vi "test.add.data.to.buffer.vi"() -> (3 "All Passed":bool=TRUE)   [LabVIEW 2020]
uses:
  data.ctl
  buffer.test.case.ctl
panel:
  in  "Test Case #12 - Buffer has 16 elements, Data has 3 elements":T1={"data.valid"=TRUE, "data"={"enabled"=[TRUE, TRUE, TRUE, FALSE, FALSE, FALSE, FALSE, FALSE], "byte"=[1, 2, 3, 4, 5, 6, 7, 0]}, "buffer"=[1234605616436508552, 48057234611961600, 0, 0, 0, 0, 0, 0, 0], "buffer.length"=16, "exp.buffer.value.1"=72623842526232576, "index 1"=2, "exp.buffer.value.2"=0, "index 2"=3, "exp.buffer.length"=19} {"exp.buffer.value.2" format="%.0x"; "index 1" format="%.0x"; "exp.buffer.value.1" format="%.0x"; "buffer" format="%.0x"; "data"."byte" format="%.0x"}
  out "Passed 12":bool=TRUE
  in  "Test Case #11 - Buffer has 16 elements, Data has 8 elements":T1={"data.valid"=TRUE, "data"={"enabled"=[TRUE, TRUE, TRUE, TRUE, TRUE, TRUE, TRUE, TRUE], "byte"=[1, 2, 3, 4, 5, 6, 7, 8]}, "buffer"=[1234605616436508552, 48057234611961600, 0, 0, 0, 0, 0, 0, 0], "buffer.length"=16, "exp.buffer.value.1"=72623859790382856, "index 1"=2, "exp.buffer.value.2"=0, "index 2"=3, "exp.buffer.length"=24} {"exp.buffer.value.2" format="%.0x"; "index 1" format="%.0x"; "exp.buffer.value.1" format="%.0x"; "buffer" format="%.0x"; "data"."byte" format="%.0x"}
  out "Passed 11":bool=TRUE
  in  "Test Case #10 - Buffer has 32 elements, Data has 8 elements":T1={"data.valid"=TRUE, "data"={"enabled"=[TRUE, TRUE, TRUE, TRUE, TRUE, TRUE, TRUE, TRUE], "byte"=[34, 255, 255, 255, 255, 255, 255, 255]}, "buffer"=[1234605616436508552, 48057234611961600, 1234605616436508552, 11024811887802974208, 0, 0, 0, 0, 0], "buffer.length"=32, "exp.buffer.value.1"=2522015791327477759, "index 1"=4, "exp.buffer.value.2"=0, "index 2"=5, "exp.buffer.length"=40} {"exp.buffer.value.2" format="%.0x"; "index 1" format="%.0x"; "exp.buffer.value.1" format="%.0x"; "buffer" format="%.0x"; "data"."byte" format="%.0x"}
  out "Passed 10":bool=TRUE
  in  "Test Case #9 - Buffer has 26 elements, Data has 1 element":T1={"data.valid"=TRUE, "data"={"enabled"=[TRUE, FALSE, FALSE, FALSE, FALSE, FALSE, FALSE, FALSE], "byte"=[34, 255, 255, 255, 255, 255, 255, 255]}, "buffer"=[1234605616436508552, 48057234611961600, 1234605616436508552, 11024811887802974208, 0, 0, 0, 0, 0], "buffer.length"=25, "exp.buffer.value.1"=11034382037011136512, "index 1"=3, "exp.buffer.value.2"=0, "index 2"=4, "exp.buffer.length"=26} {"exp.buffer.value.2" format="%.0x"; "index 1" format="%.0x"; "exp.buffer.value.1" format="%.0x"; "buffer" format="%.0x"; "data"."byte" format="%.0x"}
  out "Passed 9":bool=TRUE
  in  "Test Case #8 - Buffer has 3 elements, Data has 8 elements 2":T1={"data.valid"=TRUE, "data"={"enabled"=[TRUE, TRUE, TRUE, TRUE, TRUE, TRUE, TRUE, TRUE], "byte"=[34, 51, 68, 85, 102, 119, 136, 170]}, "buffer"=[1234605322945953792, 0, 0, 0, 0, 0, 0, 0, 0], "buffer.length"=3, "exp.buffer.value.1"=1234605469834958182, "index 1"=0, "exp.buffer.value.2"=8613321204322795520, "index 2"=1, "exp.buffer.length"=11} {"exp.buffer.value.2" format="%.0x"; "index 1" format="%.0x"; "exp.buffer.value.1" format="%.0x"; "buffer" format="%.0x"; "data"."byte" format="%.0x"}
  out "Passed 8":bool=TRUE
  in  "Test Case #7 - Buffer has 3 elements, Data has 8 elements":T1={"data.valid"=TRUE, "data"={"enabled"=[TRUE, TRUE, TRUE, TRUE, TRUE, TRUE, TRUE, TRUE], "byte"=[34, 51, 68, 85, 102, 119, 136, 170]}, "buffer"=[1234605322945953792, 0, 0, 0, 0, 0, 0, 0, 0], "buffer.length"=3, "exp.buffer.value.1"=1234605469834958182, "index 1"=0, "exp.buffer.value.2"=8613321204322795520, "index 2"=1, "exp.buffer.length"=11} {"exp.buffer.value.2" format="%.0x"; "index 1" format="%.0x"; "exp.buffer.value.1" format="%.0x"; "buffer" format="%.0x"; "data"."byte" format="%.0x"}
  out "Passed 7":bool=TRUE
  in  "Test Case #6 - Buffer has 3 elements, Data has 1 element":T1={"data.valid"=TRUE, "data"={"enabled"=[TRUE, FALSE, FALSE, FALSE, FALSE, FALSE, FALSE, FALSE], "byte"=[68, 255, 255, 255, 255, 255, 255, 255]}, "buffer"=[1234605322945953792, 0, 0, 0, 0, 0, 0, 0, 0], "buffer.length"=3, "exp.buffer.value.1"=1234605615003729920, "index 1"=0, "exp.buffer.value.2"=0, "index 2"=1, "exp.buffer.length"=4} {"exp.buffer.value.2" format="%.0x"; "index 1" format="%.0x"; "exp.buffer.value.1" format="%.0x"; "buffer" format="%.0x"; "data"."byte" format="%.0x"}
  out "Passed 6":bool=TRUE
  in  "Test Case #5 - Buffer has 1 element, Data has 8 elements":T1={"data.valid"=TRUE, "data"={"enabled"=[TRUE, TRUE, TRUE, TRUE, TRUE, TRUE, TRUE, TRUE], "byte"=[34, 51, 68, 85, 102, 119, 136, 170]}, "buffer"=[1224979098644774912, 0, 0, 0, 0, 0, 0, 0, 0], "buffer.length"=1, "exp.buffer.value.1"=1234605616436508552, "index 1"=0, "exp.buffer.value.2"=12249790986447749120, "index 2"=1, "exp.buffer.length"=9} {"exp.buffer.value.2" format="%.0x"; "index 1" format="%.0x"; "exp.buffer.value.1" format="%.0x"; "buffer" format="%.0x"; "data"."byte" format="%.0x"}
  out "Passed 5":bool=TRUE
  in  "Test #":i16=2
  in  "Override":bool
  out "Passed 4":bool=TRUE
  in  "Test Case #4 - Buffer has 1 element, Data has 7 elements":T1={"data.valid"=TRUE, "data"={"enabled"=[TRUE, TRUE, TRUE, TRUE, TRUE, TRUE, TRUE, FALSE], "byte"=[34, 51, 68, 85, 102, 119, 136, 255]}, "buffer"=[1224979098644774912, 0, 0, 0, 0, 0, 0, 0, 0], "buffer.length"=1, "exp.buffer.value.1"=1234605616436508552, "index 1"=0, "exp.buffer.value.2"=0, "index 2"=1, "exp.buffer.length"=8} {"exp.buffer.value.2" format="%.0x"; "index 1" format="%.0x"; "exp.buffer.value.1" format="%.0x"; "buffer" format="%.0x"; "data"."byte" format="%.0x"}
  out "Passed 3":bool=TRUE
  in  "Test Case #3 - Buffer has 1 element, Data has 5 elements":T1={"data.valid"=TRUE, "data"={"enabled"=[TRUE, TRUE, TRUE, TRUE, TRUE, FALSE, FALSE, FALSE], "byte"=[34, 51, 68, 85, 102, 255, 255, 255]}, "buffer"=[1224979098644774912, 0, 0, 0, 0, 0, 0, 0, 0], "buffer.length"=1, "exp.buffer.value.1"=1234605616436477952, "index 1"=0, "exp.buffer.value.2"=0, "index 2"=1, "exp.buffer.length"=6} {"exp.buffer.value.2" format="%.0x"; "index 1" format="%.0x"; "exp.buffer.value.1" format="%.0x"; "buffer" format="%.0x"; "data"."byte" format="%.0x"}
  out "Passed 2":bool=TRUE
  in  "Test Case #2 - Buffer is Empty, Data has 5 elements":T1={"data.valid"=TRUE, "data"={"enabled"=[TRUE, TRUE, TRUE, TRUE, TRUE, FALSE, FALSE, FALSE], "byte"=[17, 34, 51, 68, 85, 255, 255, 255]}, "buffer"=[0, 0, 0, 0, 0, 0, 0, 0, 0], "buffer.length"=0, "exp.buffer.value.1"=1234605616429793280, "index 1"=0, "exp.buffer.value.2"=0, "index 2"=1, "exp.buffer.length"=5} {"exp.buffer.value.2" format="%.0x"; "index 1" format="%.0x"; "exp.buffer.value.1" format="%.0x"; "buffer" format="%.0x"; "data"."byte" format="%.0x"}
  out "Passed 1":bool=TRUE
  in  "Test Case #1 - Buffer is Empty, Data has 8 elements":T1={"data.valid"=TRUE, "data"={"enabled"=[TRUE, TRUE, TRUE, TRUE, TRUE, TRUE, TRUE, TRUE], "byte"=[17, 34, 51, 68, 85, 102, 119, 136]}, "buffer"=[0, 0, 0, 0, 0, 0, 0, 0, 0], "buffer.length"=0, "exp.buffer.value.1"=1234605616436508552, "index 1"=0, "exp.buffer.value.2"=0, "index 2"=1, "exp.buffer.length"=8} {"exp.buffer.value.2" format="%.0x"; "index 1" format="%.0x"; "exp.buffer.value.1" format="%.0x"; "buffer" format="%.0x"; "data"."byte" format="%.0x"}
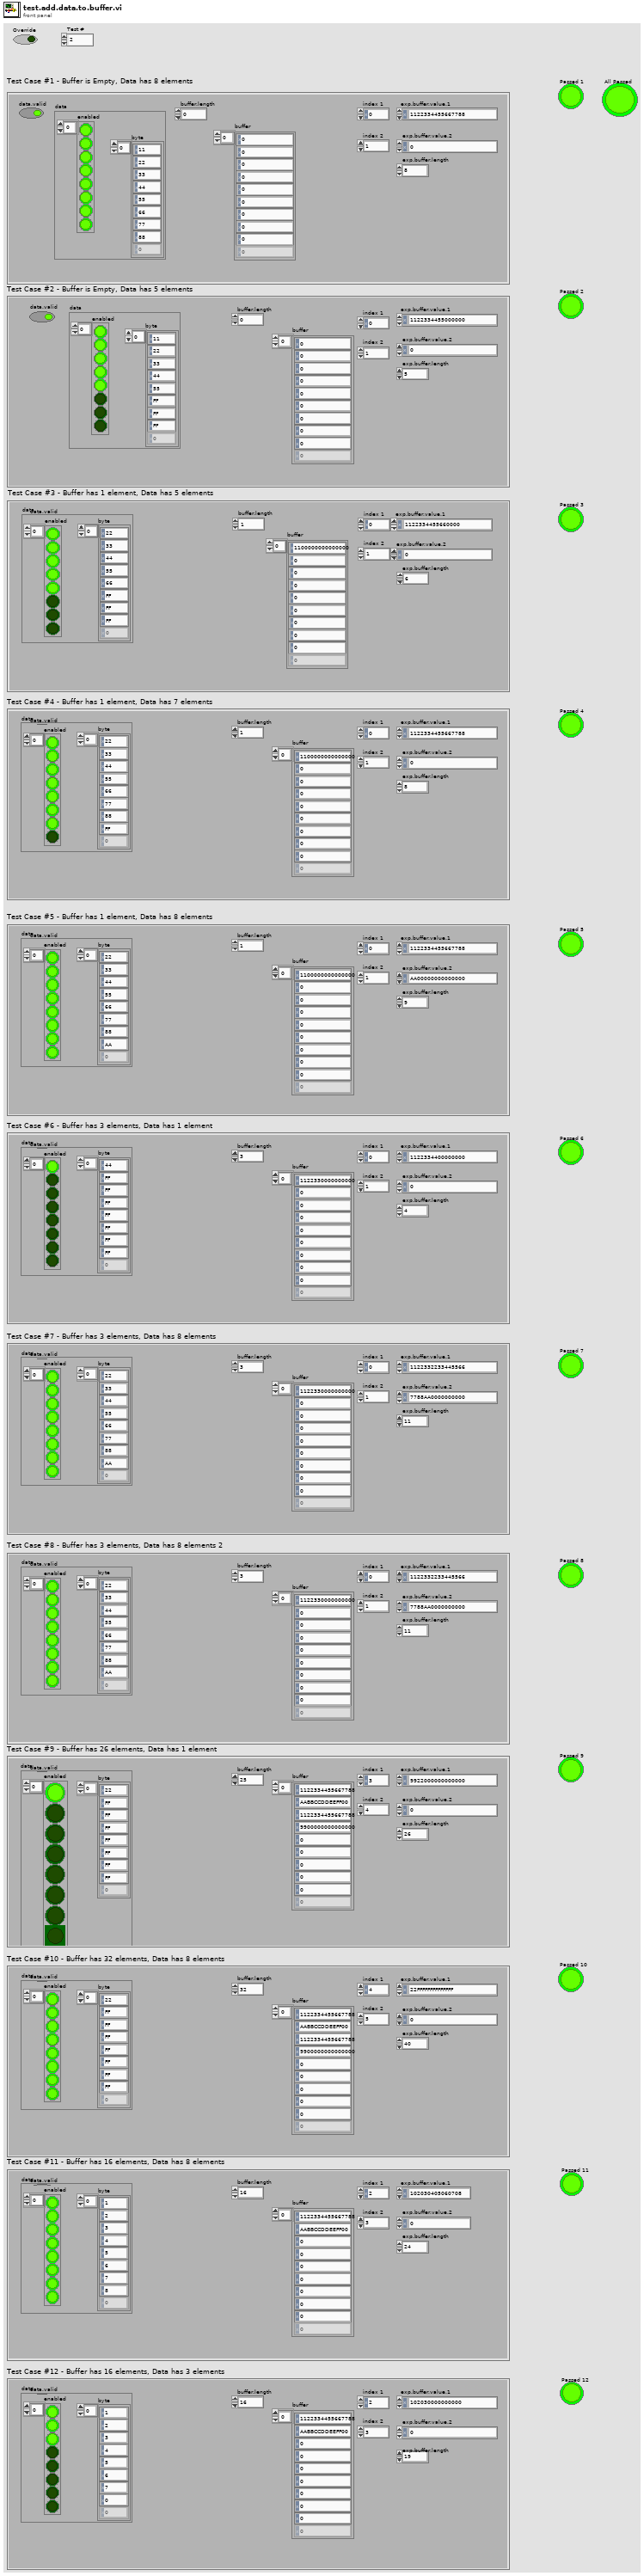
[diagram p1: front panel]
types:
  T1 = typedef "buffer.test.case.ctl" = cluster{"data.valid":bool, "data":T2, "buffer":u64[], "buffer.length":u8, "exp.buffer.value.1":u64, "index 1":i16, "exp.buffer.value.2":u64, "index 2":i16, "exp.buffer.length":u8}
  T2 = typedef "data.ctl" = cluster{"enabled":bool[], "byte":u8[]}
  T3 = typedef "niInstr Ethernet Utilities FPGA v1.lvlib/Network Data Stream.ctl" = cluster{"data":u8[], "data valid":bool, "byte enables":bool[]}
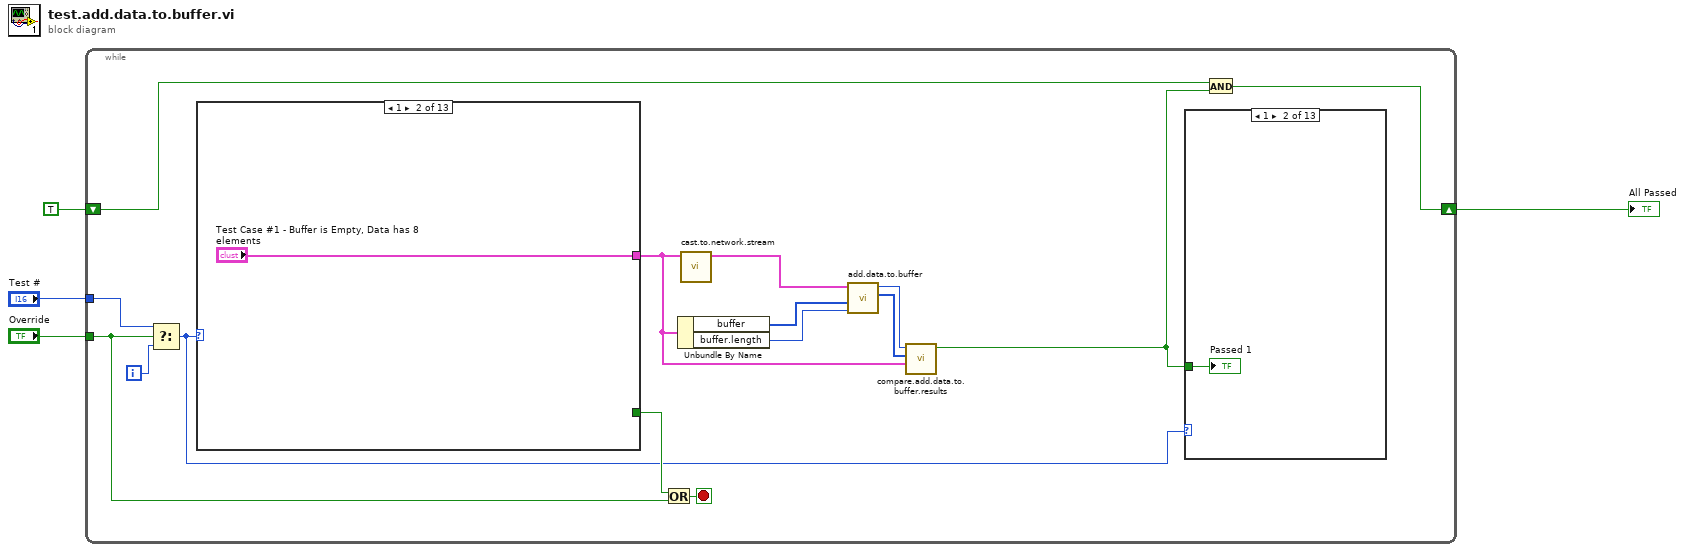
[diagram p0: block diagram]
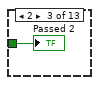
[diagram p3: hidden frame]
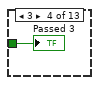
[diagram p4: hidden frame]
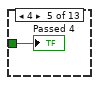
[diagram p5: hidden frame]
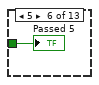
[diagram p6: hidden frame]
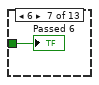
[diagram p7: hidden frame]
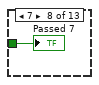
[diagram p8: hidden frame]
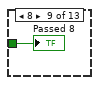
[diagram p9: hidden frame]
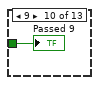
[diagram p10: hidden frame]
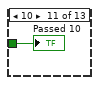
[diagram p11: hidden frame]
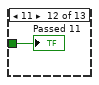
[diagram p12: hidden frame]
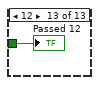
[diagram p13: hidden frame]
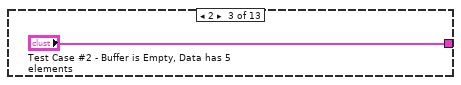
[diagram p15: hidden frame]
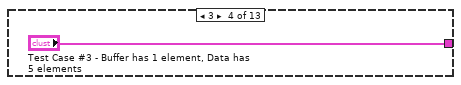
[diagram p16: hidden frame]
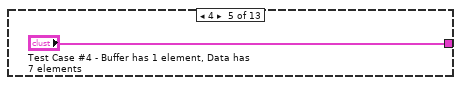
[diagram p17: hidden frame]
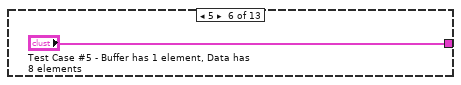
[diagram p18: hidden frame]
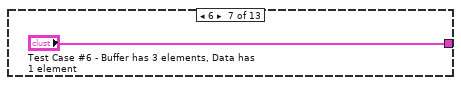
[diagram p19: hidden frame]
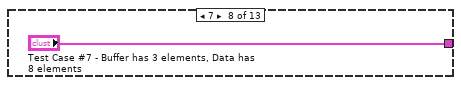
[diagram p20: hidden frame]
diagram:
  n1 = while {
    tunnel: "Test #" -> [w18]
    tunnel: "Override" -> [w15]
    shift-right: [w8] -> w4
    shift-left: TRUE -> [w5]
    i -> [w17]
    stop <- w16 stop-if-true
    n2 = Select(t=w18, s=w15, f=w17) -> (s? t:f=w9:i32)
    n3 = case shown="1" w9 {
      tunnel: [_ _ _ _ _ _ _ _ _ _ _ _ TRUE] -> w19
      tunnel: [_ "Test Case #1 - Buffer is Empty, Data has 8 elements" "Test Case #2 - Buffer is Empty, Data has 5 elements" "Test Case #3 - Buffer has 1 element, Data has 5 elements" "Test Case #4 - Buffer has 1 element, Data has 7 elements" "Test Case #5 - Buffer has 1 element, Data has 8 elements" "Test Case #6 - Buffer has 3 elements, Data has 1 element" "Test Case #7 - Buffer has 3 elements, Data has 8 elements" "Test Case #8 - Buffer has 3 elements, Data has 8 elements 2" "Test Case #9 - Buffer has 26 elements, Data has 1 element" "Test Case #10 - Buffer has 32 elements, Data has 8 elements" "Test Case #11 - Buffer has 16 elements, Data has 8 elements" "Test Case #12 - Buffer has 16 elements, Data has 3 elements"] -> w6
      frame 0, Default {
      }
      frame 1 {
      }
      frame 2 {
      }
      frame 3 {
      }
      frame 4 {
      }
      frame 5 {
      }
      frame 6 {
      }
      frame 7 {
      }
      frame 8 {
      }
      frame 9 {
      }
      frame 10 {
      }
      frame 11 {
      }
      frame 12 {
      }
    }
    n4 = Or(x=w19, y=w15) -> (x .or. y?=w16:bool)
    n5 = Unbundle By Name(w6) -> ("buffer"=w12:u64[], "buffer.length"=w11:u8)
    n6 = call "cast.to.network.stream.vi"("Test Case"=w6) -> ("network Data Stream.ctl"=w7:cluster{"reset":bool, "Data Stream":T3})  [unwired: 10 in]
    n7 = call "add.data.to.buffer.vi"("buffer.length"=w11, "buffer"=w12, "data.stream"=w7) -> ("buffer.out"=w13:u64[], "buffer.length.out"=w14:u8)  [unwired: 7 in]
    n8 = call "compare.add.data.to.buffer.results.vi"("Test Case"=w6, "buffer.out"=w13, "buffer.length.out"=w14) -> ("All Passed"=w10:bool)  [unwired: 8 in]
    n9 = case shown="1" w9 {
      tunnel: w10 -> [_ w20 w21 w22 w23 w24 w25 w26 w27 w28 w29 w30 w31]
      frame 0, Default {
      }
      frame 1 {
        "Passed 1" <- w20
      }
      frame 2 {
        "Passed 2" <- w21
      }
      frame 3 {
        "Passed 3" <- w22
      }
      frame 4 {
        "Passed 4" <- w23
      }
      frame 5 {
        "Passed 5" <- w24
      }
      frame 6 {
        "Passed 6" <- w25
      }
      frame 7 {
        "Passed 7" <- w26
      }
      frame 8 {
        "Passed 8" <- w27
      }
      frame 9 {
        "Passed 9" <- w28
      }
      frame 10 {
        "Passed 10" <- w29
      }
      frame 11 {
        "Passed 11" <- w30
      }
      frame 12 {
        "Passed 12" <- w31
      }
    }
    n10 = And(x=w5, y=w10) -> (x .and. y?=w8:bool)
  }
  "All Passed" <- w4
